vi "Decompress.vi"(9 "Active Compressed In":string[](array[string]), 11 "Trace Items In":cluster{string, bool}[](array[cluster])) -> (3 "Trace Items Out":cluster{string, bool}[](array[cluster]))   [LabVIEW 2018, in "TracerLibrary.lvlib" / "Tracer.lvclass"]
uses:
  Tracer.lvclass
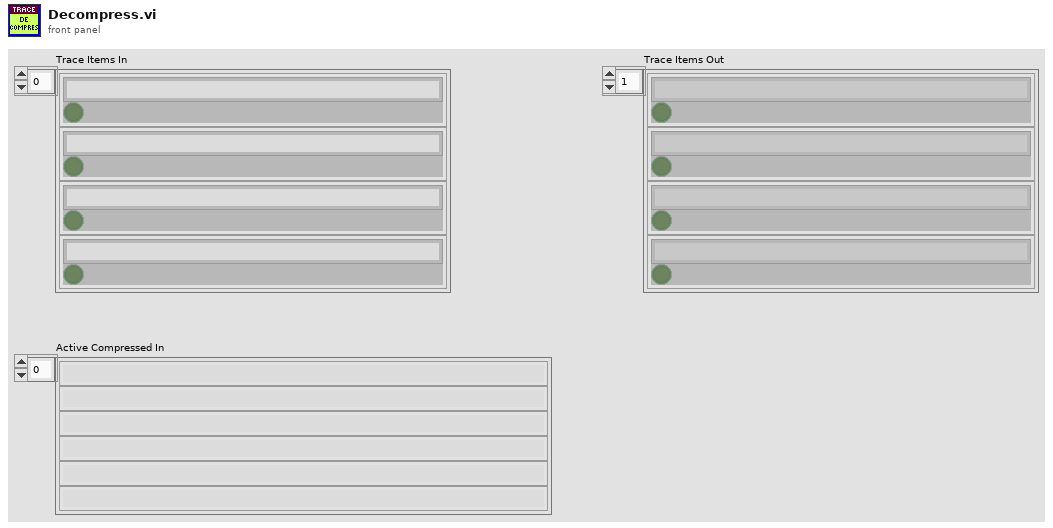
[diagram p1: front panel]
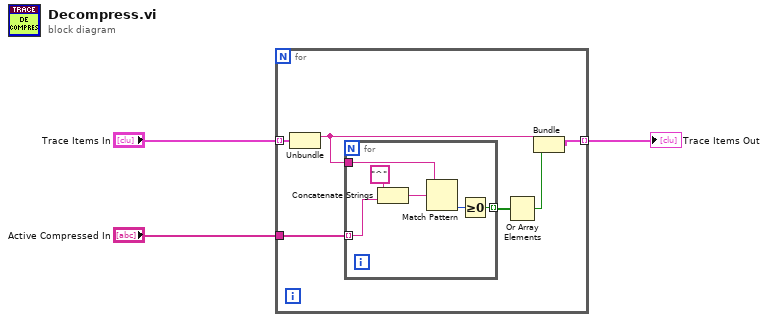
[diagram p0: block diagram]
diagram:
  n1 = for {
    tunnel: "Trace Items In" -> [w8] mode=indexing
    tunnel: "Active Compressed In" -> [w9]
    tunnel: [w4] -> w1 mode=indexing
    n2 = Unbundle(w8) -> (w6:string)  [unwired: 1 out]
    n3 = for {
      tunnel: w9 -> [w15] mode=indexing
      tunnel: w6 -> [w11]
      tunnel: [w10] -> w7 mode=indexing
      n4 = Concatenate Strings("^" ("string"), w15) -> (w13:string)
      n5 = Match Pattern(string=w11, regular expression=w13) -> (offset past match=w14:i32)  [unwired: 1 in, 3 out]
      n6 = Greater Or Equal To 0?(x=w14) -> (x >= 0?=w10:bool)
    }
    n7 = Or Array Elements(Boolean array=w7) -> (logical OR=w5:bool)
    n8 = Bundle(w6, w5) -> (w4:cluster{string, bool})  [unwired: 1 in]
  }
  "Trace Items Out" <- w1
